vi "hAdres2014.vi"(4 "error in":errorcluster, 5 "Kanal#":u8, 6 "AdressMode":enum16{"select", "oben", "unten", "keinen"}(ring), 7 "FPGA VI Reference In":refnum<k20>) -> (0 "error out":errorcluster, 3 "FPGA VI Reference Out":refnum<k20>)   [LabVIEW 2014]
doc: "Wählt je nach Auswahl alle oberen bzw unteren oder einen einzelnen Kanal aus."
uses:
  <vilib>/Utility/error.llb/Error Cluster From Error Code.vi
  <vilib>/rvi/errors/niLvFpgaAdjustHostInterfaceError.vi
  <vilib>/rvi/interface/nirviReadWriteControl/nirviReadWriteControl.xnode
  FPGA Bitfiles/W7XBolo2017_FPGATarget_fmain2014_DACRangeVoltage.lvbitx
  f_main_2014.vi
  NiFpgaLv.dll
panel:
  out "Boolean array 4":bool[](array[boolean])
  out "Boolean array 3":bool[](array[boolean])
  out "Boolean array 2":bool[](array[boolean])
  out "Boolean array":bool[](array[boolean])
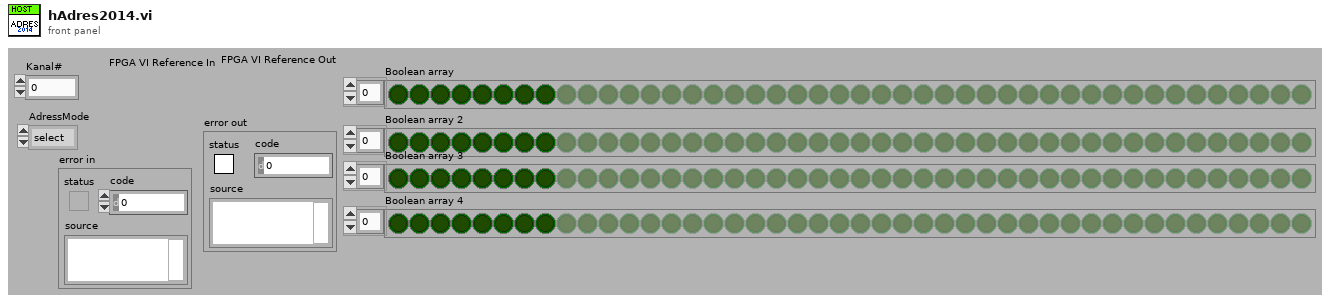
[diagram p1: front panel]
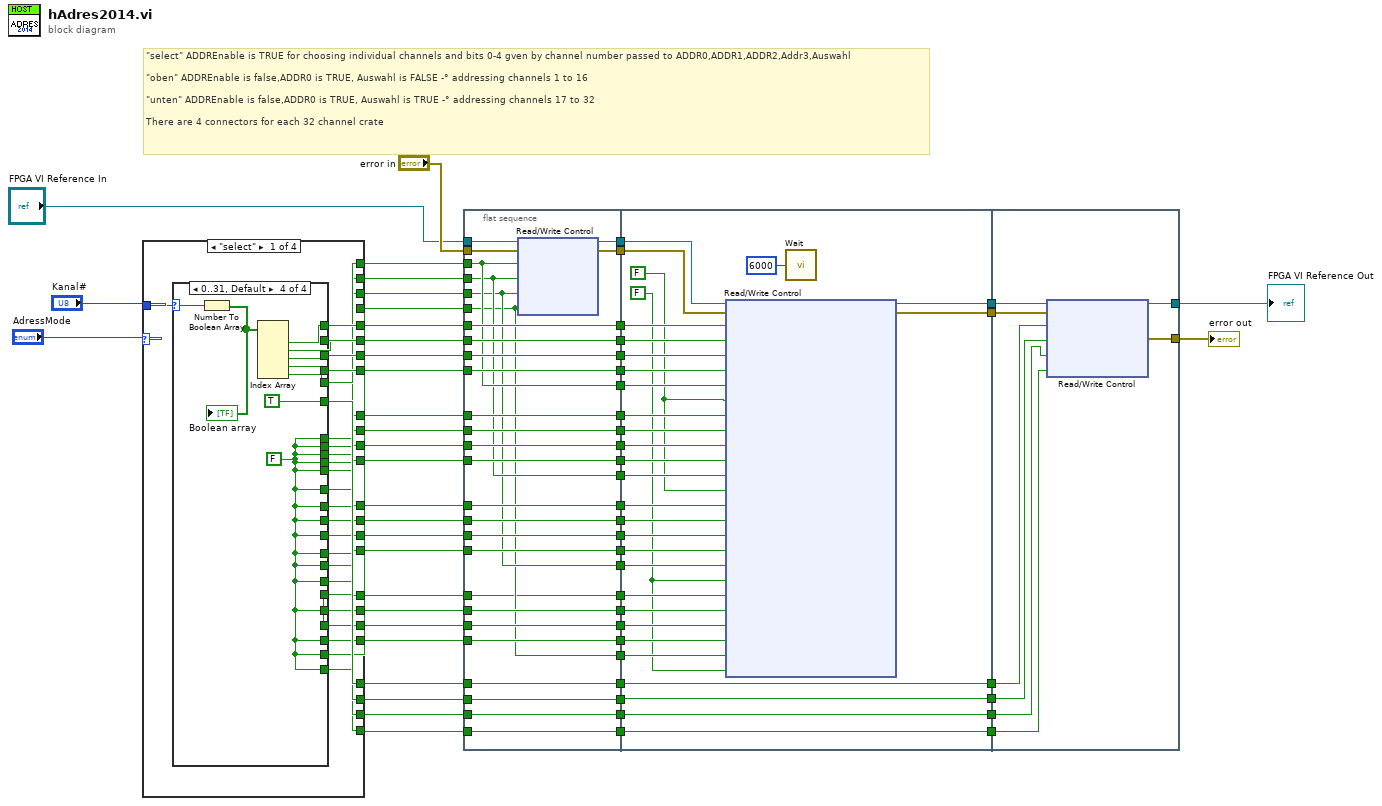
[diagram p0: block diagram]
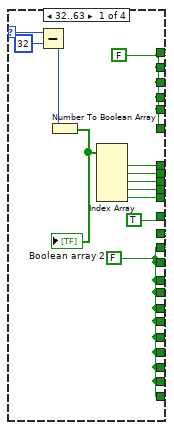
[diagram p2: hidden frame]
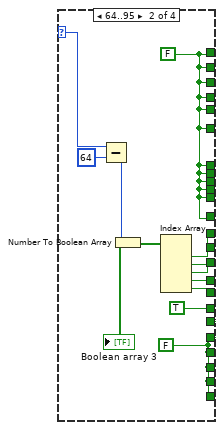
[diagram p3: hidden frame]
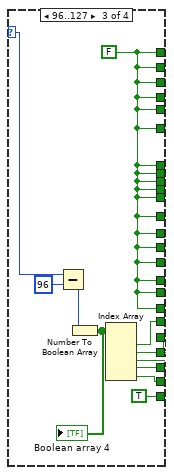
[diagram p4: hidden frame]
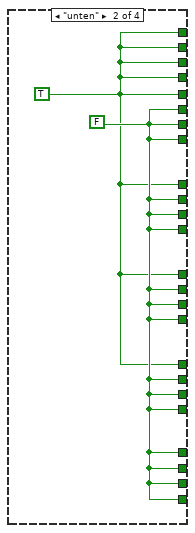
[diagram p5: hidden frame]
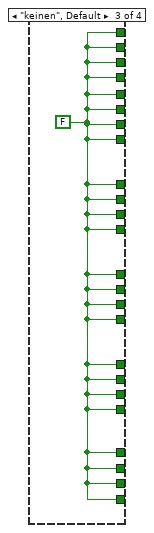
[diagram p6: hidden frame]
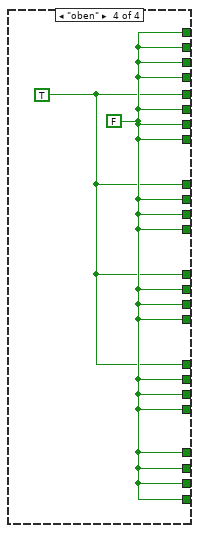
[diagram p7: hidden frame]
diagram:
  # "\"select\" ADDREnable is TRUE for choosing individual channels and bits 0-4 gven by channel number passed to ADDR0,ADDR1,ADDR2,Addr3,Auswahl\n\n\"oben\" ADDREnable is false,ADDR0 is TRUE, Auswahl is FALSE -° addressing channels 1 to 16\n\n\"unten\" ADDREnable is false,ADDR0 is TRUE, Auswahl is TRUE -° addressing channels 17 to 32\n\nThere are 4 connectors for each 32 channel crate"
  n1 = case shown="\"select\"" "AdressMode" {
    tunnel: "Kanal#" -> [w81 _ _ _]
    tunnel: [w86 w133 w134 w136] -> w61
    tunnel: [w85 w132 w134 w135] -> w60
    tunnel: [w84 w133 w134 w136] -> w59
    tunnel: [w87 w133 w134 w136] -> w58
    tunnel: [w83 w133 w134 w136] -> w57
    tunnel: [w82 w132 w134 w136] -> w1
    tunnel: [w80 w132 w134 w136] -> w2
    tunnel: [w79 w133 w134 w136] -> w52
    tunnel: [w78 w133 w134 w136] -> w3
    tunnel: [w77 w133 w134 w136] -> w53
    tunnel: [w76 w132 w134 w135] -> w54
    tunnel: [w75 w133 w134 w136] -> w51
    tunnel: [w74 w132 w134 w135] -> w45
    tunnel: [w73 w133 w134 w136] -> w46
    tunnel: [w72 w133 w134 w136] -> w47
    tunnel: [w71 w133 w134 w136] -> w48
    tunnel: [w63 w132 w134 w136] -> w49
    tunnel: [w70 w133 w134 w136] -> w50
    tunnel: [w69 w132 w134 w135] -> w41
    tunnel: [w68 w133 w134 w136] -> w40
    tunnel: [w64 w133 w134 w136] -> w39
    tunnel: [w67 w133 w134 w136] -> w42
    tunnel: [w66 w132 w134 w136] -> w43
    tunnel: [w65 w133 w134 w136] -> w44
    frame "select" {
      n2 = case shown="0..31, Default" w81 {
        selector: w81 -> [w98 w108 w119 w124]
        tunnel: [w89 w101 w112 w130] -> w87
        tunnel: [w89 w101 w112 TRUE] -> w86
        tunnel: [w89 w101 w112 w128] -> w85
        tunnel: [w89 w101 w112 w127] -> w84
        tunnel: [w89 w101 w112 w126] -> w83
        tunnel: [w89 w101 w112 w125] -> w82
        tunnel: [w95 w101 w112 w123] -> w80
        tunnel: [w94 w101 w112 w123] -> w79
        tunnel: [w93 w101 w112 w123] -> w78
        tunnel: [w92 w101 w112 w123] -> w77
        tunnel: [w91 w101 w112 w123] -> w76
        tunnel: [TRUE w101 w112 w123] -> w75
        tunnel: [w88 w107 w112 w123] -> w74
        tunnel: [w88 w106 w112 w123] -> w73
        tunnel: [w88 w105 w112 w123] -> w72
        tunnel: [w88 w104 w112 w123] -> w71
        tunnel: [w88 w103 w112 w123] -> w63
        tunnel: [w88 TRUE w112 w123] -> w70
        tunnel: [w88 w100 w118 w123] -> w69
        tunnel: [w88 w100 w117 w123] -> w68
        tunnel: [w88 w100 w115 w123] -> w67
        tunnel: [w88 w100 w114 w123] -> w66
        tunnel: [w88 w100 TRUE w123] -> w65
        tunnel: [w88 w100 w116 w123] -> w64
        frame 32..63 {
          w88 = FALSE
          w89 = FALSE
          n3 = Subtract(x=w98, y=u8 32) -> (x-y=w96:u8)
          n4 = Number To Boolean Array(number=w96) -> (Boolean array=w99:bool[])
          "Boolean array 2" <- w99
          n5 = Index Array(array=w99) -> (element #1=w91:bool, element #2=w92:bool, element #3=w93:bool, element #4=w94:bool, element #5=w95:bool)  [unwired: 5 in]
        }
        frame 64..95 {
          w100 = FALSE
          w101 = FALSE
          n6 = Subtract(x=w108, y=u8 64) -> (x-y=w109:u8)
          n7 = Number To Boolean Array(number=w109) -> (Boolean array=w111:bool[])
          "Boolean array 3" <- w111
          n8 = Index Array(array=w111) -> (element #1=w107:bool, element #2=w106:bool, element #3=w105:bool, element #4=w104:bool, element #5=w103:bool)  [unwired: 5 in]
        }
        frame 96..127 {
          w112 = FALSE
          n9 = Subtract(x=w119, y=u8 96) -> (x-y=w120:u8)
          n10 = Number To Boolean Array(number=w120) -> (Boolean array=w122:bool[])
          "Boolean array 4" <- w122
          n11 = Index Array(array=w122) -> (element #1=w118:bool, element #2=w117:bool, element #3=w116:bool, element #4=w115:bool, element #5=w114:bool)  [unwired: 5 in]
        }
        frame 0..31, Default {
          w123 = FALSE
          n12 = Number To Boolean Array(number=w124) -> (Boolean array=w131:bool[])
          "Boolean array" <- w131
          n13 = Index Array(array=w131) -> (element #1=w128:bool, element #2=w127:bool, element #3=w130:bool, element #4=w126:bool, element #5=w125:bool)  [unwired: 5 in]
        }
      }
    }
    frame "unten" {
      w133 = FALSE
      w132 = TRUE
    }
    frame "keinen", Default {
      w134 = FALSE
    }
    frame "oben" {
      w136 = FALSE
      w135 = TRUE
    }
  }
  n14 = flat-sequence {
    tunnel: w39 -> [w145]
    tunnel: w40 -> [w146]
    tunnel: w41 -> [w137]
    tunnel: w42 -> [w147]
    tunnel: w43 -> [w138]
    tunnel: w44 -> [w148]
    tunnel: w45 -> [w149]
    tunnel: w46 -> [w150]
    tunnel: w47 -> [w151]
    tunnel: w48 -> [w152]
    tunnel: w49 -> [w139]
    tunnel: w50 -> [w153]
    tunnel: w51 -> [w154]
    tunnel: w2 -> [w140]
    tunnel: w52 -> [w155]
    tunnel: w3 -> [w156]
    tunnel: w53 -> [w157]
    tunnel: w54 -> [w158]
    tunnel: "FPGA VI Reference In" -> [w159]
    tunnel: w1 -> [w141]
    tunnel: w57 -> [w160]
    tunnel: w58 -> [w161]
    tunnel: w59 -> [w162]
    tunnel: w60 -> [w163]
    tunnel: w61 -> [w164]
    tunnel: "error in" -> [w143]
    tunnel: [w142] -> w38
    tunnel: [w164] -> w37
    tunnel: [w163] -> w36
    tunnel: [w162] -> w35
    tunnel: [w161] -> w34
    tunnel: [w160] -> w33
    tunnel: [w141] -> w32
    tunnel: [w144] -> w31
    tunnel: [w158] -> w30
    tunnel: [w157] -> w29
    tunnel: [w156] -> w28
    tunnel: [w155] -> w27
    tunnel: [w140] -> w26
    tunnel: [w154] -> w25
    tunnel: [w153] -> w24
    tunnel: [w139] -> w23
    tunnel: [w152] -> w22
    tunnel: [w151] -> w21
    tunnel: [w150] -> w20
    tunnel: [w149] -> w19
    tunnel: [w148] -> w18
    tunnel: [w138] -> w17
    tunnel: [w147] -> w16
    tunnel: [w137] -> w15
    tunnel: [w146] -> w14
    tunnel: [w145] -> w13
    tunnel: w38 -> [w195]
    tunnel: w37 -> [w168]
    tunnel: w36 -> [w194]
    tunnel: w35 -> [w193]
    tunnel: w34 -> [w192]
    tunnel: w33 -> [w191]
    tunnel: w32 -> [w190]
    tunnel: w31 -> [w187]
    tunnel: w30 -> [w185]
    tunnel: w29 -> [w184]
    tunnel: w28 -> [w183]
    tunnel: w27 -> [w182]
    tunnel: w26 -> [w181]
    tunnel: w25 -> [w169]
    tunnel: w24 -> [w170]
    tunnel: w23 -> [w180]
    tunnel: w22 -> [w179]
    tunnel: w21 -> [w178]
    tunnel: w20 -> [w177]
    tunnel: w19 -> [w176]
    tunnel: w18 -> [w171]
    tunnel: w17 -> [w172]
    tunnel: w16 -> [w175]
    tunnel: w15 -> [w167]
    tunnel: w14 -> [w174]
    tunnel: w13 -> [w173]
    tunnel: [w189] -> w12
    tunnel: [w188] -> w11
    tunnel: [w171] -> w9
    tunnel: [w170] -> w8
    tunnel: [w169] -> w7
    tunnel: [w168] -> w6
    tunnel: [w200] -> w5
    tunnel: w12 -> [w203]
    tunnel: w11 -> [w202]
    tunnel: [w201] -> w10
    tunnel: w9 -> [w199]
    tunnel: w8 -> [w198]
    tunnel: w7 -> [w197]
    tunnel: w6 -> [w196]
    frame #0 {
      n15 = xnode "Read/Write Control"("FPGA VI Reference In"=w159, "error in"=w143, "C0Auswahl"=w141, "C1Auswahl"=w140, "C2Auswahl"=w139, "C3Auswahl"=w138) -> ("FPGA VI Reference Out"=w144:refnum<k20>, "error out"=w142:errorcluster)
    }
    frame #1 {
      w166 = FALSE
      w165 = FALSE
      n16 = xnode "Read/Write Control"("FPGA VI Reference In"=w187, "error in"=w195, "C0ADDR0"=w194, "C0ADDR1"=w193, "C0ADDR2"=w192, "C0ADDR3"=w191, "C0Auswahl"=w190, "C0ADDREnable"=w165, "C1ADDR0"=w185, "C1ADDR1"=w184, "C1ADDR2"=w183, "C1ADDR3"=w182, "C1Auswahl"=w181, "C1ADDREnable"=w165, "C2ADDR0"=w176, "C2ADDR1"=w177, "C2ADDR2"=w178, "C2ADDR3"=w179, "C2Auswahl"=w180, "C2ADDREnable"=w166, "C3ADDR0"=w167, "C3ADDR1"=w174, "C3ADDR2"=w173, "C3ADDR3"=w175, "C3Auswahl"=w172, "C3ADDREnable"=w166) -> ("FPGA VI Reference Out"=w189:refnum<k20>, "error out"=w188:errorcluster)
      n17 = call "Wait"("Count(uSec)"=u32 6000) -> ()  [unwired: 1 out]
    }
    frame #2 {
      n18 = xnode "Read/Write Control"("FPGA VI Reference In"=w203, "error in"=w202, "C0ADDREnable"=w196, "C1ADDREnable"=w197, "C2ADDREnable"=w198, "C3ADDREnable"=w199) -> ("FPGA VI Reference Out"=w200:refnum<k20>, "error out"=w201:errorcluster)
    }
  }
  "error out" <- w10
  "FPGA VI Reference Out" <- w5
